vi "A2 Command.vi"(8 "error in (no error)":errorcluster, 11 "DUT Serial #":i32) -> (0 "error out":errorcluster)   [LabVIEW 2015]
uses:
  RxTx/XceiverStates.ctl
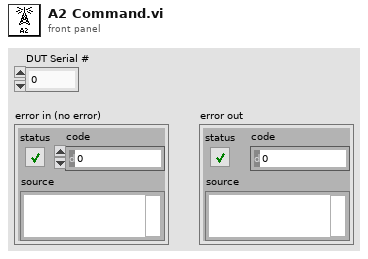
[diagram p1: front panel]
types:
  T1 = typedef "XceiverStates.ctl" = enum16{"Initialize", "Rx", "Tx", "Raw Mode", "Clear Buffer", "ClearEcho", "Read Buffer", "Close"}
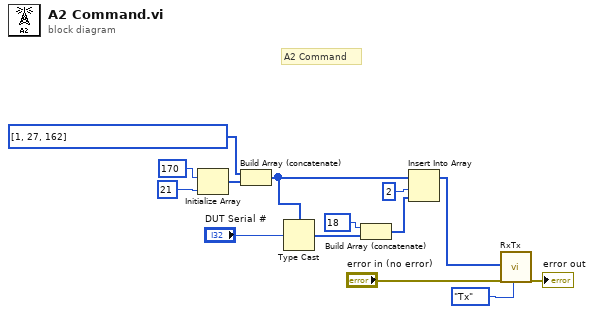
[diagram p0: block diagram]
diagram:
  # "A2 Command"
  n1 = Initialize Array(u8 170, 21 ("dimension size")) -> (w6:u8[])
  n2 = Build Array (concatenate)(u8[] [1, 27, 162] ("initialized array"), w6) -> (w5:u8[])
  n3 = Type Cast(type=w5, x="DUT Serial #") -> (*(type *) &x=w7:u8[])
  n4 = Build Array (concatenate)(u8 18, w7) -> (w3:u8[])
  n5 = Insert Into Array(array=w5, index=2, new element=w3) -> (w14:u8[])
  n6 = call "RxTx.vi"("[TxData]"=w14, "error in (no error)"="error in (no error)", "Action"=XceiverStates."Tx") -> ("error out"=→"error out":errorcluster)  [unwired: 8 in, 8 out]
